vi "Create or Replace File.vi"(8 "error in (no error)":errorcluster, 10 "Log File Base Path":path) -> (0 "error out":errorcluster, 2 "File Path":path, 3 "Refnum out":refnum<k34>)   [LabVIEW 2019, in "Logger.lvlib"]
doc: "_____\nBased on Delacor QMH Project Template 5.0.0.82."
uses:
  Logger.lvlib
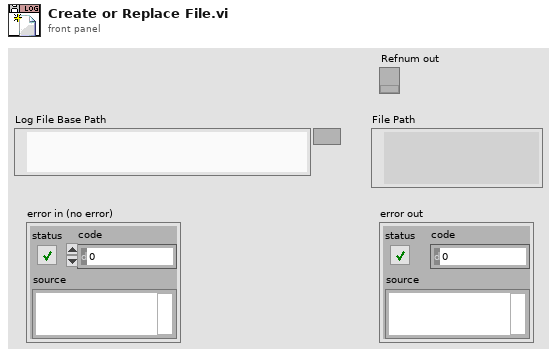
[diagram p1: front panel]
types:
  T1 = enum16{"open", "open or create", "create or replace", "create", "open (read-only)"}
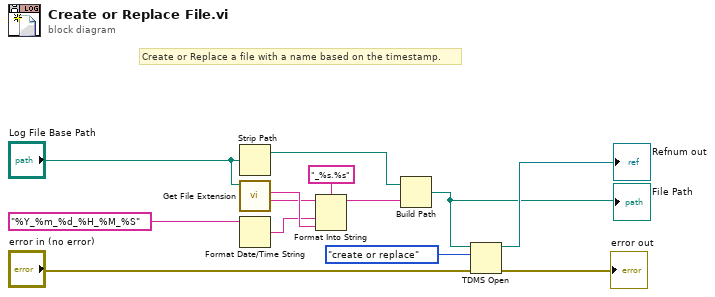
[diagram p0: block diagram]
diagram:
  # "Create or Replace a file with a name based on the timestamp."
  n1 = Strip Path(path="Log File Base Path") -> (stripped path=w5:path)  [unwired: 1 out]
  n2 = call <vilib>:"Get File Extension.vi"("file"="Log File Base Path") -> ("filename without extension"=w4:string, "lowercase file extension"=w8:string)  [unwired: 6 in, 3 out]
  n3 = Format Date/Time String(time format string (%c)="%Y_%m_%d_%H_%M_%S") -> (date/time string=w7:string)  [unwired: 2 in]
  n4 = Format Into String(format string="_%s.%s", initial string=w4, w7, w8) -> (resulting string=w9:string)  [unwired: 1 in, 1 out]
  n5 = Build Path(base path=w5, name or relative path=w9) -> (appended path=w1:path)
  "File Path" <- w1
  n6 = TDMS Open(8:"error in (no error)", 10:T1."create or replace" ("operation (0:open)"), 11:w1) -> (0:→"error out":errorcluster, 3:→"Refnum out":refnum<k34>)  [unwired: 4 in]
